vi "TL main rev B.vi"() -> ()   [LabVIEW 2014]
uses:
  boatStatus.ctl
  <vilib>/Utility/inputDevices.llb/keyboardAcquire.vi
  <vilib>/Utility/inputDevices.llb/closeKeyboard.vi
panel:
  in  "Use Laser?":bool
  out "Forebrain ACT":dbl[](array[numeric])
  in  "Tab Control":T1(tab)
  out "Image":T2(plugin-control)
  in  "stop":bool
  out "Midbrain?":bool
  in  "Manual?":bool
  out "Rudder":dbl(knob) min=-45.0 max=45.0 step=1.0 scale=-45.0..45.0
  out "Speed":dbl(knob) min=-9.0 max=9.0 step=1.0 scale=-50.0..50.0
  out "GPS":cluster{"X pos":i32, "Y pos":i32, "Heading":dbl}
  out "Power":dbl format="%#.0f"
  out "Hindbrain?":bool
  out "Forebrain?":bool
  out "Battery Dead?":bool
  out "Stuck?":bool
  in  "Battery":dbl=30000.0 format="%#_13g"
  in  "Run?":bool
  out "Complete?":bool
  out "Arbiter Graph":cluster{dbl, dbl, dbl[]}(graph)
  out "Manual\nSpeed":dbl min=-9.0 max=9.0 step=1.0
  out "Manual\nRudder":dbl min=-45.0 max=45.0 step=1.0
  out "Act Com":T3
  in  "Pool image\nfile name":string="pool image wall and buoy.png"
  in  "Boat image\nfile name":string="boat image.png"
  out "error out":errorcluster
  out "IR Sensors":T4(array[cluster])
  out "Occ Grid":u32[][](array[numeric])
  out "Forebrain Comd":T5
  out "Boat Status":T6
  out "Invalid Pos?":bool
  in  "MDF":T7(array[cluster])=[{"Type"=enum."Start", "X"=250, "Y"=250, "Speed"=0, "Behaviors"=enum."Open Water Transit"}, {"Type"=enum."Waypoint", "X"=400, "Y"=100, "Speed"=20, "Behaviors"=enum."P-Wall Follow"}, {"Type"=enum."Waypoint", "X"=250, "Y"=250, "Speed"=20, "Behaviors"=enum."Open Water Transit"}, {"Type"=enum."Waypoint", "X"=250, "Y"=400, "Speed"=20, "Behaviors"=enum."Open Water Transit"}, {"Type"=enum."Waypoint", "X"=100, "Y"=400, "Speed"=20, "Behaviors"=enum."Open Water Transit"}, {"Type"=enum."End", "X"=250, "Y"=250, "Speed"=0, "Behaviors"=enum."Open Water Transit"}]
  out "size(s)":i32
  # "ON"
  # "OFF"
  # "Boat status"
  # "In Manual mode, use the arrow keys to control the boat \nThe \"/\" centers the rudder.  Rudder is in degrees, speed in pixels/sec"
  # "To start the simulation, press the \">\" key\nin the tool bar.  Press the Manual? control to\ncontrol the boat using the keyboard.  Press\nthe Run? control to start the Mission.  When\ncomplete the Complete? indicator will light.\nIf the Run? is not pressed again, the mission\nwill start again."
  # "When the battery is dead the boat will stop.\nThe \"Power\" shows the remain battery  charge."
  # "Stuck indicates that\nthe boat is not moving."
  # "This control set the initial\nbattery power charge."
  # "This page is used to plan the mission.  The MDF, Mission Definition File, control below is used for that purpose.\n\n*  Each mission must begin with a record of type \"Start\" and end with a record of type \"End\"\n*  For the \"Start\" and \"End\" records the remaining entries have no impact.\n*  For the \"Waypoint\" records you must set a position for the waypoint, a speed, and a behavior.\n*  Any number of records may be used.\n*  The simulation will place a \"yellow\" marker at the local of each waypoint include.\n*  If you declare unused records type \"End\" they will not be include in the simulation"
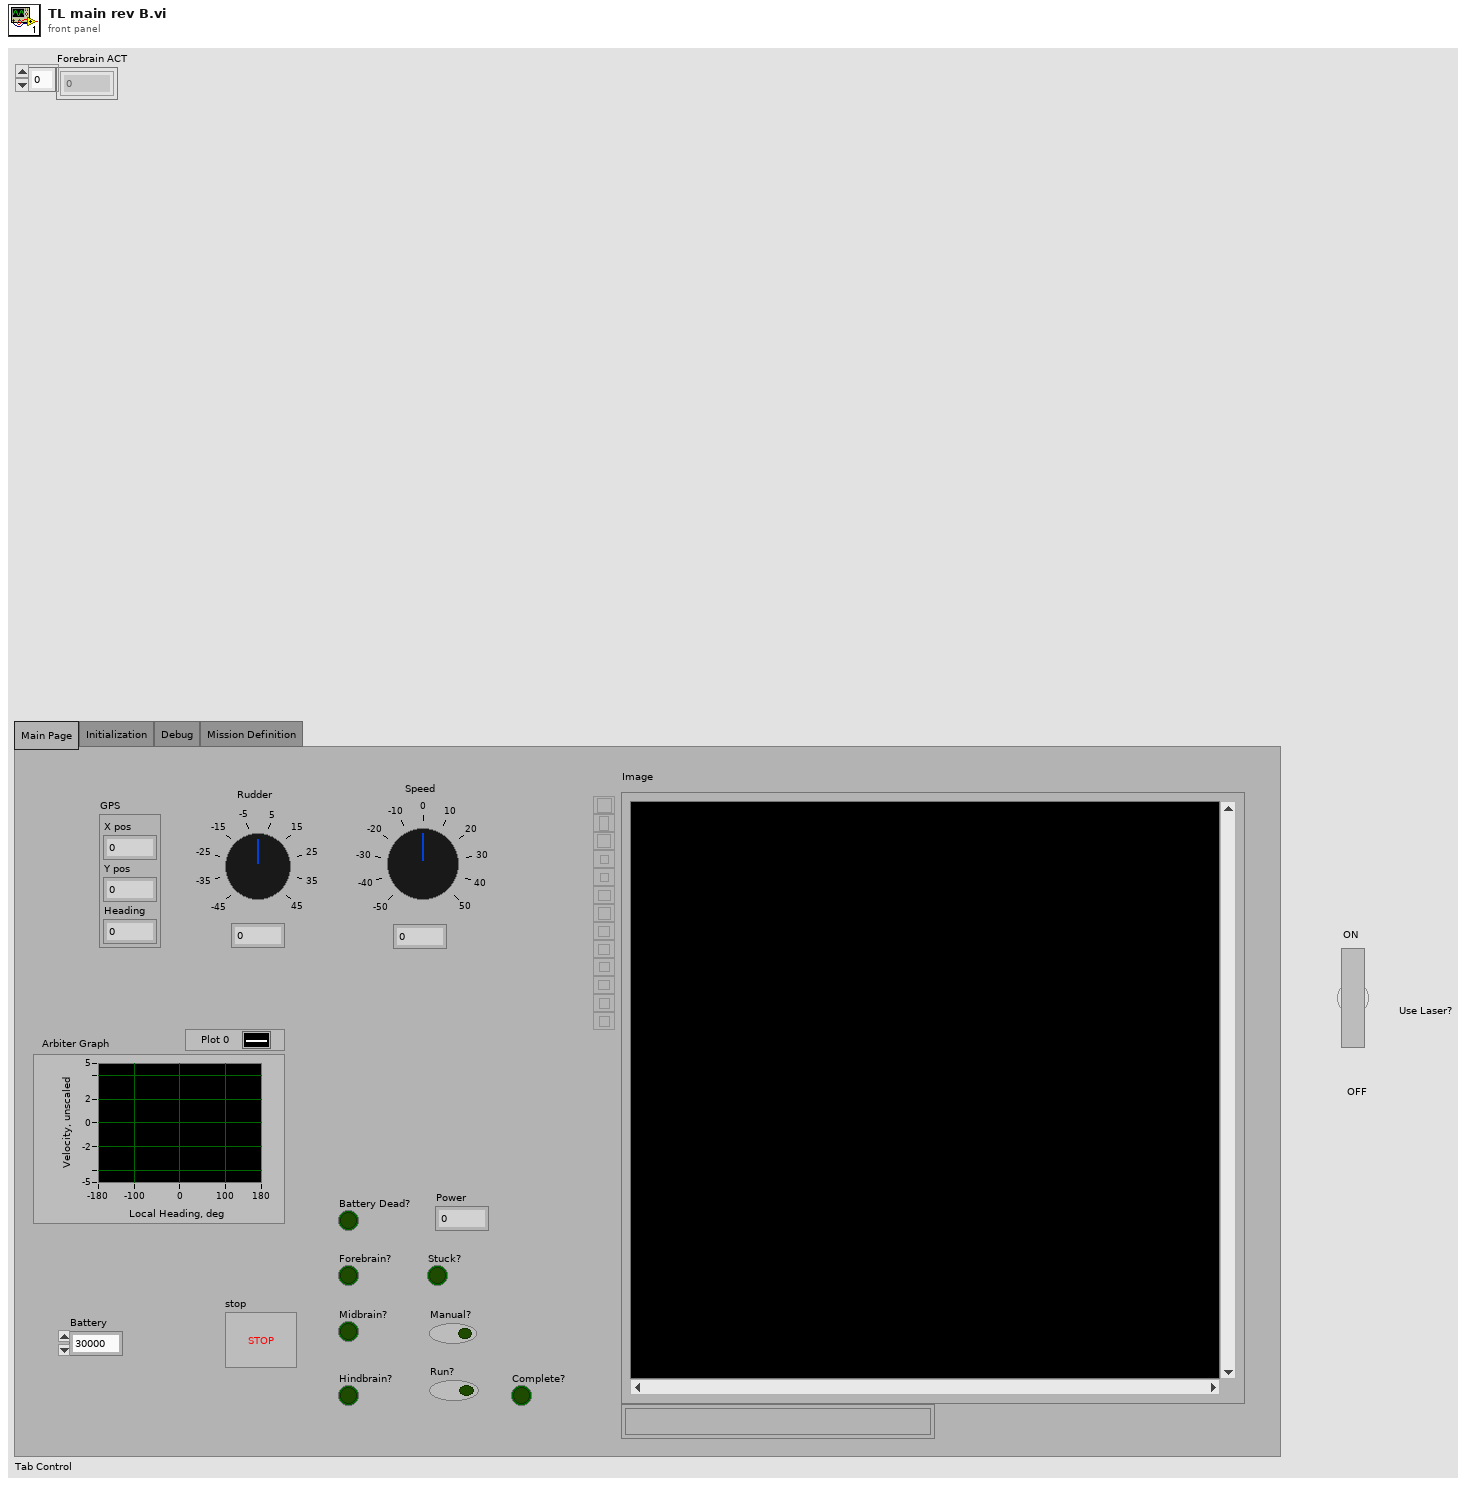
[diagram p1: front panel]
types:
  T1 = enum32{"Main Page", "Initialization", "Debug", "Mission Definition"}
  T2 = typedef "IMAQ Image.ctl" = refnum<image>
  T3 = cluster{"Desired Local\nHeading":dbl, "Desired\nSpeed":dbl}
  T4 = cluster{"Name":string, "Angle":dbl, "Distance":dbl}[]
  T5 = cluster{"Behaviors":enum16{"Open Water Transit", "P-Wall Follow", "S-Wall Follow", "Get Unstuck"}, "Behavior\nVelocity":dbl}
  T6 = typedef "boatStatus.ctl" = cluster{"GPS":cluster{"X pos":i32, "Y pos":i32, "Heading":dbl}, "IR Sensors":cluster{"Name":string, "Angle":dbl, "Distance":dbl}[], "Power":dbl}
  T7 = cluster{"Type":enum16{"Start", "Waypoint", "End"}, "X":i32, "Y":i32, "Speed":i32, "Behaviors":enum16{"Open Water Transit", "P-Wall Follow", "S-Wall Follow", "Get Unstuck"}}[]
  T8 = enum16{"Open Water Transit", "P-Wall Follow", "S-Wall Follow", "Get Unstuck"}
  T9 = typedef "Image Type" = u32
  T10 = typedef "sensorsSTD.ctl" = cluster{"Name":string, "Angle":dbl, "Distance":dbl}[]
  T11 = cluster{"Obs Avoid Array":dbl[], "P-Wall Array":dbl[], "S-Wall Array":dbl[], "Unstuck Array":dbl[]}
  T12 = cluster{"Behaviors":enum16{"Open Water Transit", "P-Wall Follow", "S-Wall Follow", "Get Unstuck"}, dbl}
  T13 = enum16{"0", "1", "2", "3", "4", "5", "6", "7", "8", "9", "A", "B", "C", "D", "E", "F", "G", "H", "I", "J", "K", "L", "M", "N", "O", "P", "Q", "R", "S", "T", "U", "V", "W", "X", "Y", "Z", "F1", "F2", "F3", "F4", "F5", "F6", "F7", "F8", "F9", "F10", "F11", "F12", "F13", "F14", "F15", "ADD", "BACK", "BACKSLASH", "CAPITAL", "COMMA", "DECIMAL", "DELETE", "DIVIDE", "DOWN", "END", "EQUALS", "ESCAPE", "GRAVE (`)", "HOME", "INSERT", "LBRACKET", "LCONTROL", "LEFT", "L ALT", "LSHIFT", "LWIN", "MINUS", "MULTIPLY", "NEXT", "NUMLOCK", "NUMPAD_0", "NUMPAD_1", "NUMPAD_2", "NUMPAD_3", "NUMPAD_4", "NUMPAD_5", "NUMPAD_6", "NUMPAD_7", "NUMPAD_8", "NUMPAD_9", "PAUSE", "PERIOD", "PRIOR (PG UP)", "RBRACKET", "RCONTROL", "RETURN", "RIGHT", "R ALT", "RSHIFT", "RWIN", "SCROLL", "SEMICOLON", "SLASH", "SPACE", "SUBTRACT", "TAB", "UP", "ENTER (num pad)", "' (quote)"}[]
  T14 = enum16{"0", "1", "2", "3", "4", "5", "6", "7", "8", "9", "A", "B", "C", "D", "E", "F", "G", "H", "I", "J", "K", "L", "M", "N", "O", "P", "Q", "R", "S", "T", "U", "V", "W", "X", "Y", "Z", "F1", "F2", "F3", "F4", "F5", "F6", "F7", "F8", "F9", "F10", "F11", "F12", "F13", "F14", "F15", "ADD", "BACK", "BACKSLASH", "CAPITAL", "COMMA", "DECIMAL", "DELETE", "DIVIDE", "DOWN", "END", "EQUALS", "ESCAPE", "GRAVE (`)", "HOME", "INSERT", "LBRACKET", "LCONTROL", "LEFT", "L ALT", "LSHIFT", "LWIN", "MINUS", "MULTIPLY", "NEXT", "NUMLOCK", "NUMPAD_0", "NUMPAD_1", "NUMPAD_2", "NUMPAD_3", "NUMPAD_4", "NUMPAD_5", "NUMPAD_6", "NUMPAD_7", "NUMPAD_8", "NUMPAD_9", "PAUSE", "PERIOD", "PRIOR (PG UP)", "RBRACKET", "RCONTROL", "RETURN", "RIGHT", "R ALT", "RSHIFT", "RWIN", "SCROLL", "SEMICOLON", "SLASH", "SPACE", "SUBTRACT", "TAB", "UP", "ENTER (num pad)", "' (quote)"}
  T15 = cluster{"Device Out":i32, "Engaged?":bool, "error out":errorcluster}
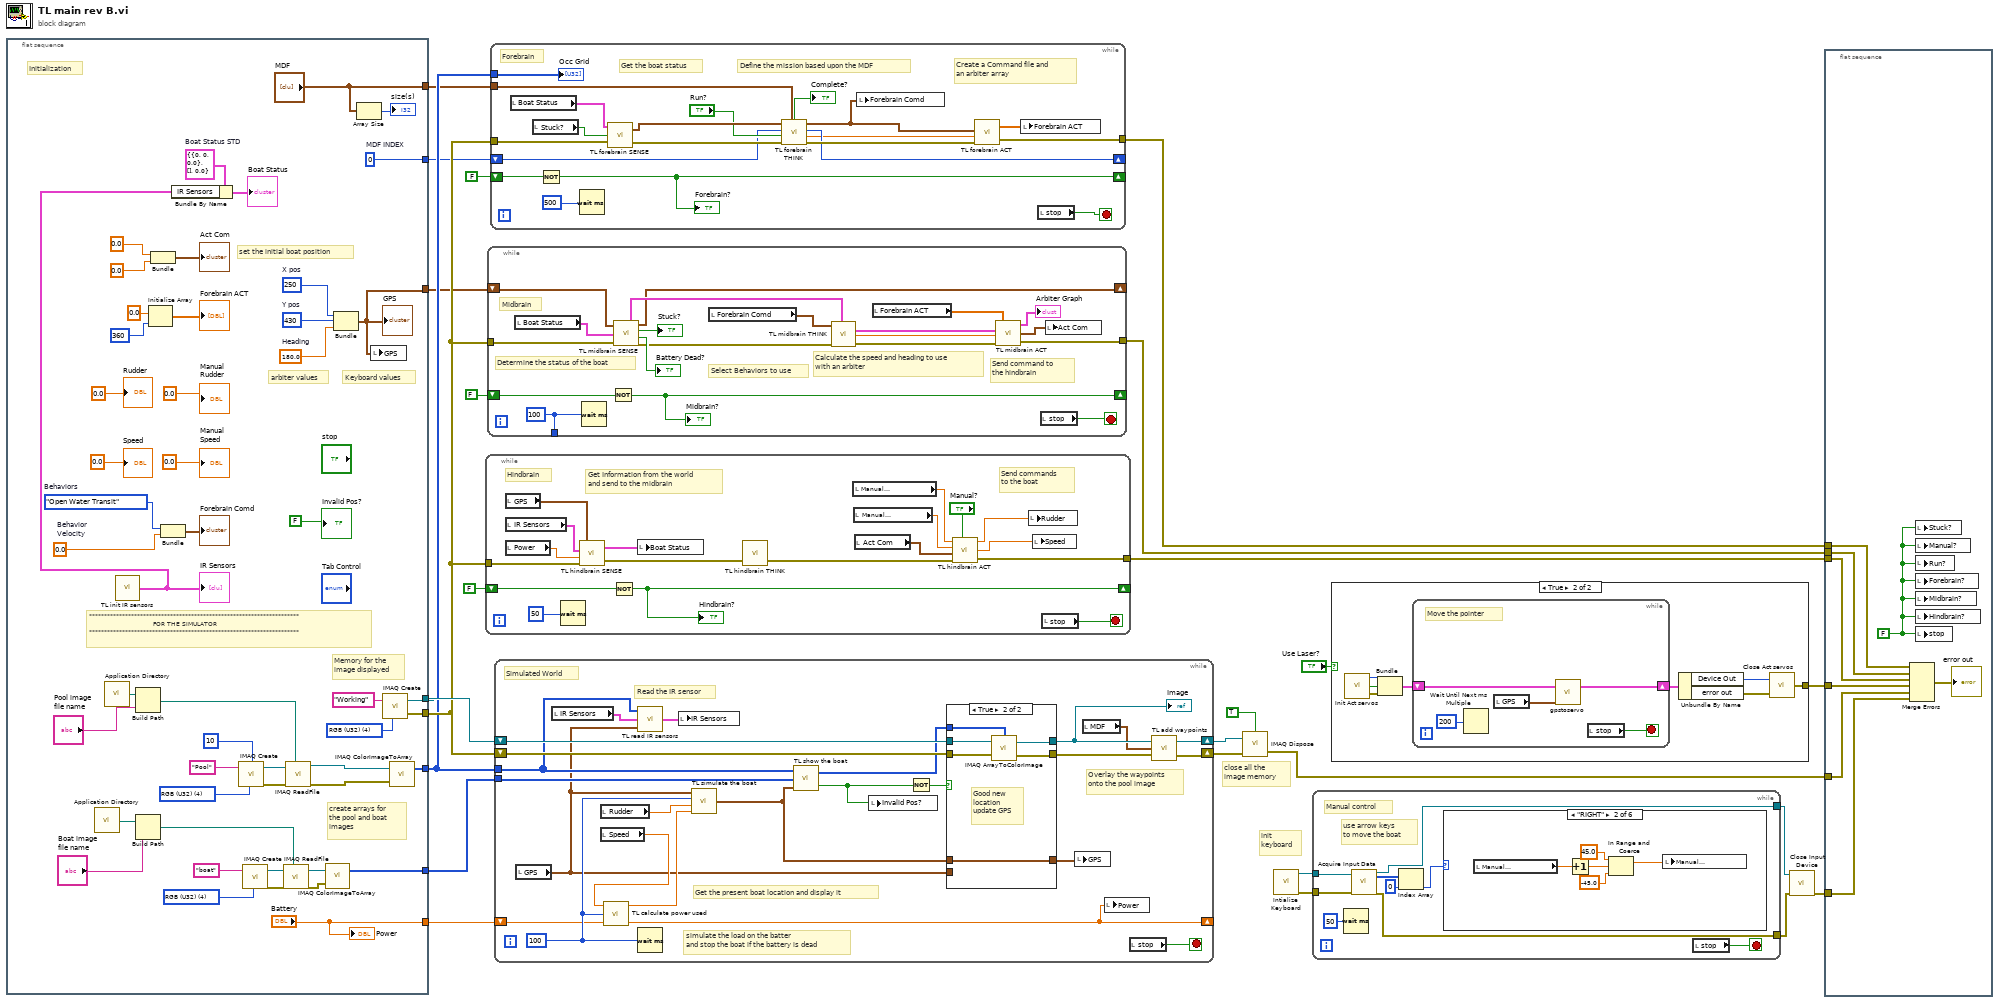
[diagram p0: block diagram]
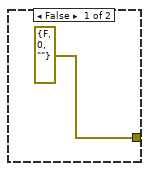
[diagram p2: hidden frame]
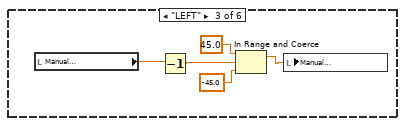
[diagram p4: hidden frame]
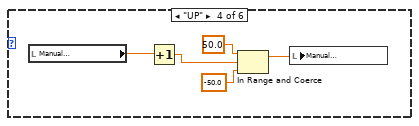
[diagram p5: hidden frame]
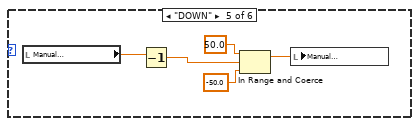
[diagram p6: hidden frame]
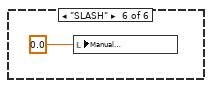
[diagram p7: hidden frame]
diagram:
  # "init\nkeyboard"
  # "close all the\nimage memory"
  n1 = flat-sequence {
    tunnel: [w64] -> w25
    tunnel: [w63] -> w13
    tunnel: [w60] -> w15
    tunnel: [w59] -> w24
    tunnel: ["Battery"] -> w17
    tunnel: [w26] -> w12
    tunnel: ["MDF"] -> w11
    tunnel: [w40] -> w10
    frame #0 {
      w29 = T6 {"GPS"={"X pos"=0, "Y pos"=0, "Heading"=0.0}, "IR Sensors"=[], "Power"=0.0}  # Boat Status STD
      w40 = 0  # MDF INDEX
      w44 = 0.0  # Behavior Velocity
      w38 = T8."Open Water Transit"  # Behaviors
      w62 = T9 4 items=["Grayscale (U8)", "Grayscale (I16)", "Grayscale (SGL)", "Complex (CSG)", "RGB (U32)", "HSL (U32)", "RGB (U64)", "Grayscale (U16)"] ("Image Type")
      w68 = T9 4 items=["Grayscale (U8)", "Grayscale (I16)", "Grayscale (SGL)", "Complex (CSG)", "RGB (U32)", "HSL (U32)", "RGB (U64)", "Grayscale (U16)"] ("Image Type")
      w72 = T9 4 items=["Grayscale (U8)", "Grayscale (I16)", "Grayscale (SGL)", "Complex (CSG)", "RGB (U32)", "HSL (U32)", "RGB (U64)", "Grayscale (U16)"] ("Image Type")
      w57 = 430  # Y pos
      w56 = 250  # X pos
      w55 = 180.0  # Heading
      # "**********************************************************************\n                                FOR THE SIMULATOR\n**********************************************************************"
      # "Initialization"
      # "Keyboard values"
      # "arbiter values"
      # "Memory for the\nimage displayed"
      # "create arrays for\nthe pool and boat\nimages"
      # "set the initial boat position"
      n2 = call <vilib>:"Application Directory.vi"() -> ("Application Directory"=w32:path)
      n3 = call <vilib>:"Application Directory.vi"() -> ("Application Directory"=w33:path)
      n4 = call "TL init IR sensors.vi"() -> ("IR Sensors"=w28:T4)  [unwired: 1 in]
      "IR Sensors" <- w28
      n5 = Build Path(base path=w32, name or relative path="Boat image\nfile name") -> (appended path=w30:path)
      n6 = Build Path(base path=w33, name or relative path="Pool image\nfile name") -> (appended path=w35:path)
      n7 = Initialize Array(0.0 ("element"), 360 ("dimension size")) -> (→"Forebrain ACT":dbl[])
      n8 = Bundle(0.0, 0.0) -> (→"Act Com":cluster{dbl, dbl})  [unwired: 1 in]
      n9 = Bundle("Behaviors"=w38, "Behavior\nVelocity"=w44) -> (→"Forebrain Comd":T5)  [unwired: 1 in]
      n10 = Bundle By Name(cluster=w29, "IR Sensors"=w28) -> (→"Boat Status":T6)
      n11 = call "IMAQ Create"("Border Size"=10, "Image Name"="Pool", "Image Type"=w72) -> ("New Image"=w74:T2, "error out"=w73:errorcluster)  [unwired: 2 in]
      n12 = call "IMAQ Create"("Image Name"="boat", "Image Type"=w68) -> ("New Image"=w70:T2, "error out"=w69:errorcluster)  [unwired: 3 in]
      n13 = call "IMAQ ReadFile"("File Path"=w30, "error in (no error)"=w69, "Image"=w70) -> ("error out"=w66:errorcluster, "Image Out"=w65:T2)  [unwired: 4 in, 3 out]
      n14 = call "IMAQ ReadFile"("File Path"=w35, "error in (no error)"=w73, "Image"=w74) -> ("error out"=w49:errorcluster, "Image Out"=w50:T2)  [unwired: 4 in, 3 out]
      n15 = call "IMAQ ColorImageToArray"("Image"=w65, "error in (no error)"=w66) -> ("Image Pixels (U32)"=w64:u32[][])  [unwired: 2 in, 2 out]
      n16 = Bundle("X pos"=w56, "Y pos"=w57, "Heading"=w55) -> (w26:cluster{"X pos":i32, "Y pos":i32, "Heading":dbl})  [unwired: 1 in]
      "GPS" <- w26
      n17 = Array Size(array="MDF") -> (size(s)=→"size(s)":i32)
      n18 = local write "GPS"(w26) -> ()
      n19 = call "IMAQ Create"("Image Name"="Working", "Image Type"=w62) -> ("New Image"=w59:T2, "error out"=w60:errorcluster)  [unwired: 3 in]
      n20 = call "IMAQ ColorImageToArray"("Image"=w50, "error in (no error)"=w49) -> ("Image Pixels (U32)"=w63:u32[][])  [unwired: 2 in, 2 out]
      "Invalid Pos?" <- FALSE
      "Manual\nRudder" <- 0.0
      "Manual\nSpeed" <- 0.0
      "Rudder" <- 0.0
      "Speed" <- 0.0
      "Power" <- "Battery"
    }
  }
  n21 = while {
    tunnel: w15 -> [w84]
    tunnel: [w85] -> w6
    shift-right: [w79] -> _
    shift-left: FALSE -> [w80]
    stop <- w93 stop-if-true
    # "Send commands\nto the boat"
    # "Get Information from the world\nand send to the midbrain"
    # "Hindbrain"
    n22 = local read "GPS"() -> (w77:cluster{"X pos":i32, "Y pos":i32, "Heading":dbl})
    n23 = local read "IR Sensors"() -> (w83:T4)
    n24 = local read "Power"() -> (w78:dbl)
    n25 = Wait (ms)(milliseconds to wait=u32 50) -> ()  [unwired: 1 out]
    n26 = call "TL hindbrain SENSE.vi"("error in"=w84, "Power in"=w78, "IR Sensors"=w83, "GPS"=w77) -> ("error out"=w82:errorcluster, "Boat Status Init"=w76:T6)
    n27 = Not(x=w80) -> (.not. x?=w79:bool)
    "Hindbrain?" <- w79
    n28 = local write "Boat Status"(w76) -> ()
    n29 = call "TL hindbrain THINK.vi"("error in"=w82) -> ("error out"=w81:errorcluster)  [unwired: 2 in]
    n30 = local read "Manual\nRudder"() -> (w91:dbl)
    n31 = local read "Manual\nSpeed"() -> (w92:dbl)
    n32 = local read "Act Com"() -> (w86:T3)
    n33 = call "TL hindbrain ACT.vi"("Manual\nRudder"=w91, "Manual\nSpeed"=w92, "Act Com"=w86, "error in"=w81, "Manual?"="Manual?") -> ("Rudder"=w90:dbl, "Speed"=w89:dbl, "error out"=w85:errorcluster)
    n34 = local write "Rudder"(w90) -> ()
    n35 = local write "Speed"(w89) -> ()
    n36 = local read "stop"() -> (w93:bool)
  }
  n37 = while {
    shift-right: [w98] -> _
    shift-left: FALSE -> [w112]
    tunnel: w15 -> [w111]
    tunnel: [w103] -> w7
    shift-right: [w94] -> _
    shift-left: w12 -> [w110]
    tunnel: [w96] -> _
    stop <- w113 stop-if-true
    w96 = u32 100 ("milliseconds to wait")
    # "Send command to \nthe hindbrain"
    # "Calculate the speed and heading to use\nwith an arbiter"
    # "Select Behaviors to use"
    # "Determine the status of the boat"
    # "Midbrain"
    n38 = local read "Boat Status"() -> (w97:T6)
    n39 = Wait (ms)(milliseconds to wait=w96) -> ()  [unwired: 1 out]
    n40 = Not(x=w112) -> (.not. x?=w98:bool)
    "Midbrain?" <- w98
    n41 = call "TL midbrain SENSE.vi"("Last location"=w110, "Boat Status"=w97, "error in"=w111) -> ("Last location out"=w94:cluster{"X pos":i32, "Y pos":i32, "Heading":dbl}, "Stuck?"=→"Stuck?":bool, "Battery\nDead?"=→"Battery Dead?":bool, "error out"=w107:errorcluster, "IR Sensors"=w95:T10)
    n42 = local read "Forebrain Comd"() -> (w100:T5)
    n43 = call "TL midbrain THINK.vi"("Forebrain Comd"=w100, "error in"=w107, "IR Sensors"=w95) -> ("Behavior arrays"=w104:T11, "Behavior\nVelocity OUT"=w101:dbl, "error out"=w106:errorcluster)  [unwired: 2 in]
    n44 = local read "Forebrain ACT"() -> (w102:dbl[])
    n45 = call "TL midbrain ACT.vi"("error in"=w106, "Behavior\nVelocity"=w101, "Behavior arrays"=w104, "Forebrain ACT"=w102) -> ("error out"=w103:errorcluster, "Act Com"=w108:T3, "Waveform Graph"=→"Arbiter Graph":cluster{dbl, dbl, dbl[]})
    n46 = local read "stop"() -> (w113:bool)
    n47 = local write "Act Com"(w108) -> ()
  }
  n48 = while {
    tunnel: w15 -> [w130]
    shift-right: [w116] -> _
    shift-left: FALSE -> [w117]
    tunnel: [w126] -> w8
    tunnel: w13 -> [w131]
    tunnel: w11 -> [w121]
    shift-right: [w123] -> _
    shift-left: w10 -> [w119]
    stop <- w132 stop-if-true
    # "Create a Command file and \nan arbiter array"
    # "Define the mission based upon the MDF"
    # "Get the boat status"
    # "Forebrain"
    n49 = local read "Boat Status"() -> (w114:T6)
    n50 = local read "Stuck?"() -> (w129:bool)
    n51 = Not(x=w117) -> (.not. x?=w116:bool)
    "Forebrain?" <- w116
    n52 = Wait (ms)(milliseconds to wait=u32 500) -> ()  [unwired: 1 out]
    n53 = call "TL forebrain SENSE.vi"("error in"=w130, "Stuck?"=w129, "Boat Status"=w114) -> ("error out"=w128:errorcluster, "GPS"=w124:cluster{"X pos":i32, "Y pos":i32, "Heading":dbl})
    n54 = call "TL forebrain THINK.vi"("MDF"=w121, "error in"=w128, "Run?"="Run?", "MDF index"=w119, "GPS"=w124) -> ("error out"=w127:errorcluster, "local Steering\nangle"=w122:dbl, "MDF Index out"=w123:i32, "Behaviors out"=w115:T12, "Complete?"=→"Complete?":bool)
    n55 = local write "Forebrain Comd"(w115) -> ()
    n56 = call "TL forebrain ACT.vi"("error in"=w127, "local Steering\nangle"=w122, "Behaviors in"=w115) -> ("error out"=w126:errorcluster, "Forebrain ACT"=w125:dbl[])  [unwired: 1 in]
    n57 = local write "Forebrain ACT"(w125) -> ()
    n58 = local read "stop"() -> (w132:bool)
    "Occ Grid" <- w131
  }
  n59 = while {
    tunnel: w25 -> [w140]
    tunnel: w13 -> [w141]
    shift-right: [w146] -> w22
    shift-left: w15 -> [w156]
    shift-right: [w147] -> w21
    shift-left: w24 -> [w155]
    shift-right: [w135] -> _
    shift-left: w17 -> [w143]
    stop <- w154 stop-if-true
    w144 = u32 100 ("milliseconds to wait")
    # "Simulated World"
    # "simulate the load on the batter\nand stop the boat if the battery is dead"
    # "Overlay the waypoints\nonto the pool image"
    # "Get the present boat location and display it"
    # "Read the IR sensor"
    n60 = local read "GPS"() -> (w136:cluster{"X pos":i32, "Y pos":i32, "Heading":dbl})
    n61 = local read "IR Sensors"() -> (w151:T4)
    n62 = local read "Rudder"() -> (w153:dbl)
    n63 = local read "Speed"() -> (w145:dbl)
    n64 = call "TL calculate power used.vi"("Power in"=w143, "Loop Time"=w144, "Speed"=w145) -> ("Power out"=w135:dbl, "Speed out"=w142:dbl)  [unwired: 1 in]
    n65 = call "TL read IR sensors.vi"("GPS"=w136, "IR Sensors"=w151, "Pool image\nPixels (U32)"=w141) -> ("IR Sensors out"=w150:T4)
    n66 = Wait (ms)(milliseconds to wait=w144) -> ()  [unwired: 1 out]
    n67 = local write "IR Sensors"(w150) -> ()
    n68 = call "TL simulate the boat.vi"("Boat Speed\npixels/sec"=w142, "Rudder"=w153, "Loop time"=w144, "GPS"=w136) -> ("GPS out"=w137:cluster{"X pos":i32, "Y pos":i32, "Heading":dbl})
    n69 = call "TL show the boat.vi"("GPS"=w137, "Boat array"=w140, "Pool array"=w141) -> ("Invalid Pos?"=w138:bool, "Pool out"=w139:u32[][])
    n70 = local write "Invalid Pos?"(w138) -> ()
    n71 = Not(x=w138) -> (.not. x?=w157:bool)
    n72 = case shown="True" w157 {
      tunnel: w156 -> [w159 w166]
      tunnel: [w159 w165] -> w149
      tunnel: w155 -> [w160 w164]
      tunnel: [w160 w163] -> w148
      tunnel: w139 -> [_ w162]
      tunnel: w136 -> [w158 _]
      tunnel: w137 -> [_ w161]
      tunnel: [w158 w161] -> w152
      frame False {
        # "invalid position\nshow the old one\nboat hit a thing"
      }
      frame True {
        # "Good new \nlocation\nupdate GPS"
        n73 = call "IMAQ ArrayToColorImage"("Image Pixels (U32)"=w162, "Image"=w164, "error in (no error)"=w166) -> ("Image Out"=w163:T2, "error out"=w165:errorcluster)  [unwired: 2 in]
      }
    }
    "Image" <- w148
    n74 = local write "GPS"(w152) -> ()
    n75 = local read "MDF"() -> (w134:T7)
    n76 = local write "Power"(w135) -> ()
    n77 = local read "stop"() -> (w154:bool)
    n78 = call "TL add waypoints.vi"("error in"=w149, "MDF"=w134, "Image In"=w148) -> ("error out"=w146:errorcluster, "Image Out"=w147:T2)
  }
  n79 = call "IMAQ Dispose"("All Images? (No)"=TRUE, "Image"=w21, "error in (no error)"=w22) -> ("error out"=w5:errorcluster)  [unwired: 3 in]
  n80 = call <vilib>:"Intialize Keyboard.vi"() -> ("error out"=w19:errorcluster, "device ID"=w18:refnum<k1>)  [unwired: 10 in]
  n81 = while {
    tunnel: w19 -> [w173]
    tunnel: w18 -> [w172]
    tunnel: [w168] -> w3
    tunnel: [w167] -> w1
    stop <- w174 stop-if-true
    # "Manual control"
    # "use arrow keys\nto move the boat"
    n82 = Wait (ms)(milliseconds to wait=u32 50) -> ()  [unwired: 1 out]
    n83 = call-poly <vilib>:"Acquire Input Data.vi"("device ID"=w172, "error in (no error)"=w173) -> ("device ID"=w167:refnum<k1>, "keys pressed"=w171:T13, "error out"=w168:errorcluster)  [unwired: 15 in]
    n84 = Index Array(array=w171, index=0) -> (element=w169:T14)
    n85 = case shown="\"RIGHT\"" w169 {
      frame "0", Default {
      }
      frame "RIGHT" {
        n86 = local read "Manual\nRudder"() -> (w180:dbl)
        n87 = Increment(x=w180) -> (x+1=w179:dbl)
        n88 = In Range and Coerce(upper limit=45.0, x=w179, lower limit=-45.0) -> (coerced(x)=w178:dbl)  [unwired: 1 out]
        n89 = local write "Manual\nRudder"(w178) -> ()
      }
      frame "LEFT" {
        n90 = local read "Manual\nRudder"() -> (w185:dbl)
        n91 = Decrement(x=w185) -> (x-1=w182:dbl)
        n92 = In Range and Coerce(upper limit=45.0, x=w182, lower limit=-45.0) -> (coerced(x)=w181:dbl)  [unwired: 1 out]
        n93 = local write "Manual\nRudder"(w181) -> ()
      }
      frame "UP" {
        n94 = local read "Manual\nSpeed"() -> (w190:dbl)
        n95 = Increment(x=w190) -> (x+1=w187:dbl)
        n96 = In Range and Coerce(upper limit=50.0, x=w187, lower limit=-50.0) -> (coerced(x)=w186:dbl)  [unwired: 1 out]
        n97 = local write "Manual\nSpeed"(w186) -> ()
      }
      frame "DOWN" {
        n98 = local read "Manual\nSpeed"() -> (w195:dbl)
        n99 = Decrement(x=w195) -> (x-1=w192:dbl)
        n100 = In Range and Coerce(upper limit=50.0, x=w192, lower limit=-50.0) -> (coerced(x)=w191:dbl)  [unwired: 1 out]
        n101 = local write "Manual\nSpeed"(w191) -> ()
      }
      frame "SLASH" {
        n102 = local write "Manual\nRudder"(0.0) -> ()
      }
    }
    n103 = local read "stop"() -> (w174:bool)
  }
  n104 = case shown="True" "Use Laser?" {
    tunnel: [errorcluster {"status"=FALSE, "code"=0, "source"=""} ("error out") w205] -> w4
    frame False {
    }
    frame True {
      n105 = call "Init Act servos.vi"() -> ("Device Out"=w204:i32, "Engaged?"=w203:bool, "error out"=w202:errorcluster)  [unwired: 1 in]
      n106 = Bundle("Device Out"=w204, "Engaged?"=w203, "error out"=w202) -> (w201:T15)  [unwired: 1 in]
      n107 = while {
        shift-right: [w206] -> w200
        shift-left: w201 -> [w208]
        stop <- w209 stop-if-true
        # "Move the pointer"
        n108 = Wait Until Next ms Multiple(millisecond multiple=u32 200) -> ()  [unwired: 1 out]
        n109 = local read "GPS"() -> (w207:cluster{"X pos":i32, "Y pos":i32, "Heading":dbl})
        n110 = call "gpstoservo.vi"("GPS Input"=w207, "Servo In Cluster"=w208) -> ("Servo Out Cluster"=w206:T15)  [unwired: 1 in]
        n111 = local read "stop"() -> (w209:bool)
      }
      n112 = Unbundle By Name(w200) -> ("Device Out"=w198:i32, "error out"=w199:errorcluster)
      n113 = call "Close Act servos.vi"("error in"=w199, "Device In"=w198) -> ("error out"=w205:errorcluster)
    }
  }
  n114 = call-poly <vilib>:"Close Input Device.vi"("error in (no error)"=w3, "device ID"=w1) -> ("error out"=w2:errorcluster)  [unwired: 8 in]
  n115 = flat-sequence {
    tunnel: w2 -> [w211]
    tunnel: w8 -> [w216]
    tunnel: w7 -> [w215]
    tunnel: w6 -> [w214]
    tunnel: w5 -> [w213]
    tunnel: w4 -> [w212]
    frame #0 {
      w218 = FALSE ("stop")
      n116 = Merge Errors(w216, w215, w214, w212, w213, w211) -> (→"error out":errorcluster)
      n117 = local write "Stuck?"(w218) -> ()
      n118 = local write "Manual?"(w218) -> ()
      n119 = local write "Run?"(w218) -> ()
      n120 = local write "Forebrain?"(w218) -> ()
      n121 = local write "Midbrain?"(w218) -> ()
      n122 = local write "Hindbrain?"(w218) -> ()
      n123 = local write "stop"(w218) -> ()
    }
  }
